vi "APU 1.4 Read Outputs.vi"(5 "degrees of 1 crank u16":dbl, 6 "max deviation angle":dbl, 7 "degrees of 1 cycle u16":dbl, 8 "error in (no error)":errorcluster, 9 "Device outputs in":dbl[](array[numeric]), 10 "output reference in":T1, 11 "FIFO indexes.outputs":T2) -> (0 "error out":errorcluster, 1 "Device outputs out":dbl[](array[numeric]), 2 "output reference out":T1)   [LabVIEW 2019, in "Engine Simulation Toolkit Engine.lvlib"]
uses:
  Engine Simulation Toolkit Engine.lvlib
  APU 1.0 Output Ref.ctl
  <vilib>/Utility/error.llb/Error Cluster From Error Code.vi
  <vilib>/rvi/errors/niLvFpgaAdjustHostInterfaceError.vi
  <vilib>/rvi/interface/nirviReadWriteControl/nirviReadWriteControl.xnode
  NiFpgaLv.dll
  <vilib>/rvi/interface/Simulation/niFpgaSimulationCallBeginRW.vi
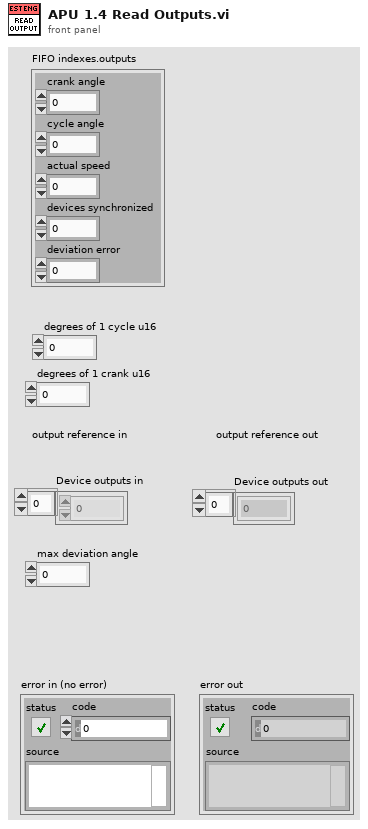
[diagram p1: front panel]
types:
  T1 = typedef "Engine Simulation Toolkit Engine.lvlib/APU 1.0 Output Ref.ctl" = refnum<k20>
  T2 = cluster{"crank angle":i32, "cycle angle":i32, "actual speed":i32, "devices synchronized":i32, "deviation error":i32}
  T3 = cluster{"crank":u16, "cycle":u16, "actual speed":fxp<+/-,23,2>}
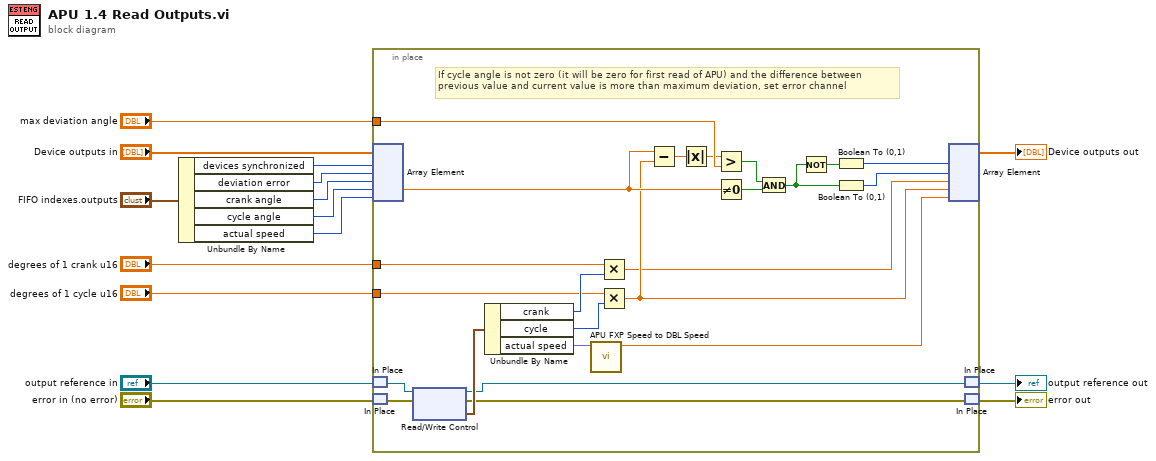
[diagram p0: block diagram]
diagram:
  n1 = Unbundle By Name("FIFO indexes.outputs") -> ("devices synchronized"=w5:i32, "deviation error"=w4:i32, "crank angle"=w3:i32, "cycle angle"=w2:i32, "actual speed"=w1:i32)
  n2 = in-place {
    in-place-border: "degrees of 1 crank u16" -> [w30]
    in-place-border: "degrees of 1 cycle u16" -> [w29]
    in-place-border: "max deviation angle" -> [w27]
    # "If cycle angle is not zero (it will be zero for first read of APU) and the difference between\nprevious value and current value is more than maximum deviation, set error channel"
    n3 = in-place-array #1("Device outputs in", w5, w4, w3, w2, w1) -> (w22:dbl)  [unwired: 4 out]
    n4 = in-place-match #2("output reference in") -> (w37:T1)
    n5 = in-place-match #3("error in (no error)") -> (w38:errorcluster)
    n6 = xnode "Read/Write Control"("FPGA VI Reference In"=w37, "error in"=w38) -> ("FPGA VI Reference Out"=w35:T1, "error out"=w34:errorcluster, "Value"=w36:T3)
    n7 = Unbundle By Name(w36) -> ("crank"=w32:u16, "cycle"=w31:u16, "actual speed"=w33:fxp<+/-,23,2>)
    n8 = call "APU FXP Speed to DBL Speed.vi"("FXP speed"=w33) -> ("DBL speed"=w21:dbl)  [unwired: 10 in]
    n9 = Multiply(x=w30, y=w32) -> (x*y=w19:dbl)
    n10 = Multiply(x=w29, y=w31) -> (x*y=w20:dbl)
    n11 = Subtract(x=w22, y=w20) -> (x-y=w28:dbl)
    n12 = Absolute Value(x=w28) -> (abs(x)=w16:dbl)
    n13 = Greater?(x=w16, y=w27) -> (0:w26:bool)
    n14 = Not Equal To 0?(x=w22) -> (x != 0?=w25:bool)
    n15 = And(x=w26, y=w25) -> (x .and. y?=w24:bool)
    n16 = Not(x=w24) -> (.not. x?=w23:bool)
    n17 = Boolean To (0,1)(Boolean=w23) -> (0, 1=w17:i16)
    n18 = Boolean To (0,1)(Boolean=w24) -> (0, 1=w18:i16)
    n19 = in-place-array #1(w17, w18, w19, w20, w21) -> (→"Device outputs out":dbl[])  [unwired: 5 out]
    n20 = in-place-match #2(w35) -> (→"output reference out":T1)
    n21 = in-place-match #3(w34) -> (→"error out":errorcluster)
  }
